vi "Reorder Steps.vi"(8 "error in (no error)":errorcluster, 10 "New Order":i32[](array[numeric]), 11 "Macro in":refnum<class "Macro.lvclass">) -> (0 "error out":errorcluster, 3 "Macro out":refnum<class "Macro.lvclass">)   [LabVIEW 2020, in "MacroAssert.lvlib" / "Macro.lvclass"]
uses:
  Macro.lvclass
  Macro.lvclass/Macro.ctl
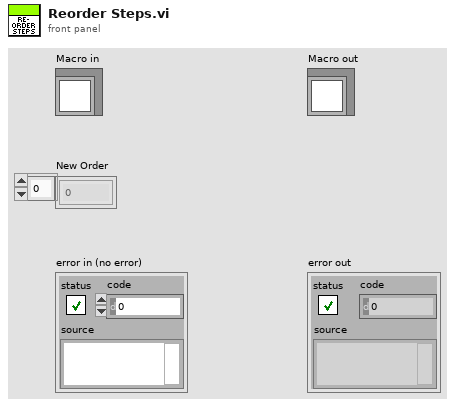
[diagram p1: front panel]
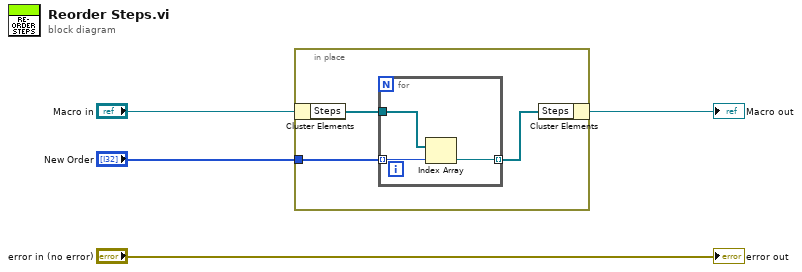
[diagram p0: block diagram]
diagram:
  n1 = in-place {
    in-place-border: "New Order" -> [w6]
    n2 = in-place-cluster #1("Macro in") -> ("Steps"=w7:refnum<class "Step.lvclass">[])
    n3 = for {
      tunnel: w7 -> [w10]
      tunnel: w6 -> [w9] mode=indexing
      tunnel: [w8] -> w5 mode=indexing
      n4 = Index Array(array=w10, index=w9) -> (element=w8:refnum<class "Step.lvclass">)
    }
    n5 = in-place-cluster #1("Steps"=w5) -> (→"Macro out":refnum<class "Macro.lvclass">)
  }
  "error out" <- "error in (no error)"
